vi "Read File Transfer Behavior.lvclass.vi"(8 "error in (no error)":errorcluster, 11 "[Test Case] Put and Get file in":refnum<class "[Test Case] Put and Get file.lvclass">) -> (0 "error out":errorcluster, 2 "RT Management.lvlib:File Transfer Behavior.lvclass":refnum<class "File Transfer Behavior.lvclass">, 3 "[Test Case] Put and Get file out":refnum<class "[Test Case] Put and Get file.lvclass">)   [LabVIEW 2015, in "Tests.lvlib" / "[Test Case] Put and Get file.lvclass"]
uses:
  [Test Case] Put and Get file.lvclass
  classes/File Transfer Behavior/File Transfer Behavior.lvclass
  [Test Case] Put and Get file.lvclass/[Test Case] Put and Get file.ctl
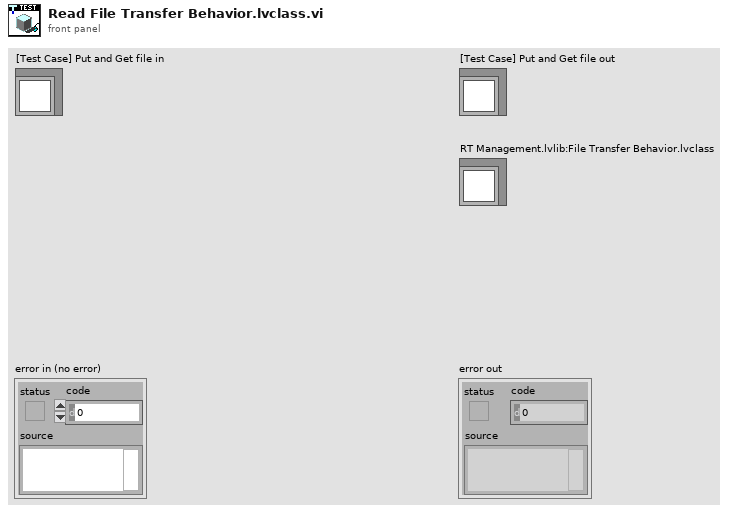
[diagram p1: front panel]
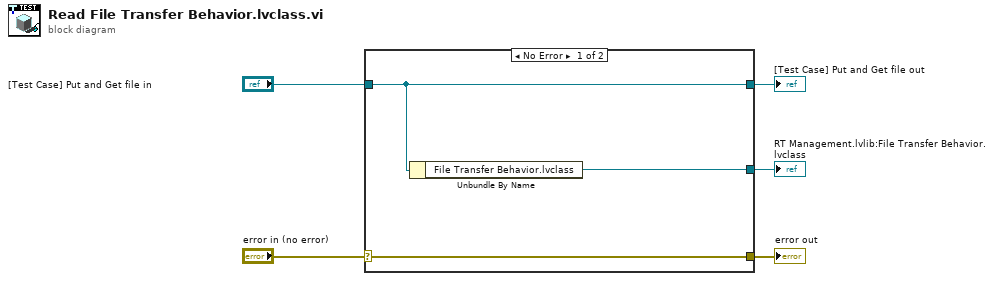
[diagram p0: block diagram]
diagram:
  n1 = case shown="No Error" "error in (no error)" {
    selector: "error in (no error)" -> [w8 w9]
    tunnel: [w8 w9] -> w4
    tunnel: [w7 w10] -> w2
    tunnel: "[Test Case] Put and Get file in" -> [w7 w10]
    tunnel: [w6 _] -> w1
    frame No Error {
      n2 = Unbundle By Name(w7) -> ("File Transfer Behavior.lvclass"=w6:refnum<class "File Transfer Behavior.lvclass">)
    }
    frame Error {
    }
  }
  "error out" <- w4
  "[Test Case] Put and Get file out" <- w2
  "RT Management.lvlib:File Transfer Behavior.lvclass" <- w1
